vi "ConvertVariantToString.vi"(8 "error in":errorcluster, 10 "Variant":variant) -> (0 "error out":errorcluster, 1 "Array of VData":variant[](array[variant]), 2 "Variant dup":variant, 3 "String":string)   [LabVIEW 2012, in "Tree Tools.lvlib" / "Tree Tag Class.lvclass"]
uses:
  Tree Tag Class.lvclass
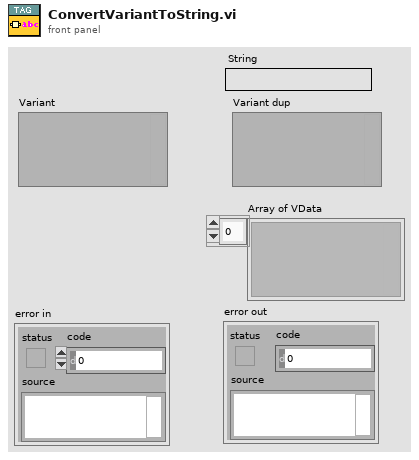
[diagram p1: front panel]
types:
  T1 = typedef "Type Descriptor Enumeration__ogtk.ctl" = enum8{"<Null>", "I8", "I16", "I32", "I64", "U8", "U16", "U32", "U64", "SGL", "DBL", "EXT", "CSG", "CDB", "CXT", "0x0F", "0x10", "0x11", "0x12", "0x13", "0x14", "Enum U8", "Enum U16", "Enum U32", "Enum U64", "SGL PQ", "DBL PQ", "EXT PQ", "CSG PQ", "CDB PQ", "CXT PQ", "0x1F", "0x20", "Boolean", "0x22", "0x23", "0x24", "0x25", "0x26", "0x27", "0x28", "0x29", "0x2A", "0x2B", "0x2C", "0x2D", "0x2E", "0x2F", "String", "0x31", "Path", "Pict", "0x34", "0x35", "0x36", "DAQ", "0x38", "0x39", "0x3A", "0x3B", "0x3C", "0x3D", "0x3E", "0x3F", "Array", "0x41", "0x42", "0x43", "0x44", "0x45", "0x46", "0x47", "0x48", "0x49", "0x4A", "0x4B", "0x4C", "0x4D", "0x4E", "0x4F", "Cluster", "0x51", "0x52", "Variant", "Waveform", "0x55", "0x56", "0x57", "0x58", "0x59", "0x5A", "0x5B", "0x5C", "0x5D", "0x5E", "0x5F", "0x60", "0x61", "0x62", "0x63", "0x64", "0x65", "0x66", "0x67", "0x68", "0x69", "0x6A", "0x6B", "0x6C", "0x6D", "0x6E", "0x6F", "Refnum"}
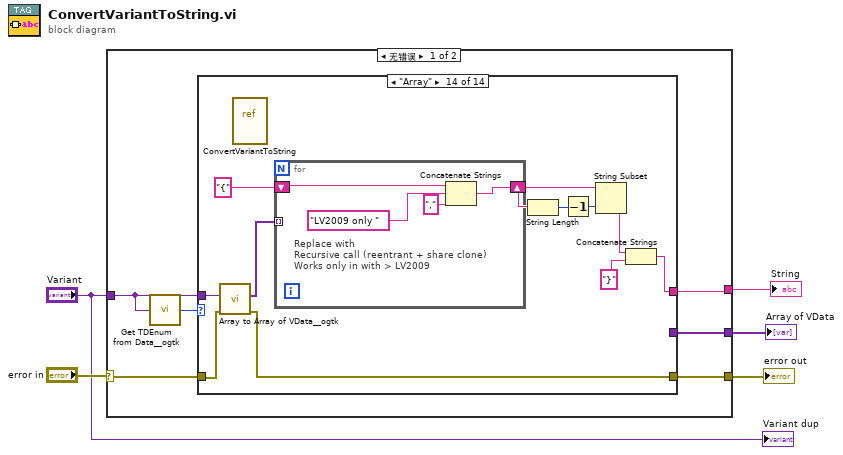
[diagram p0: block diagram]
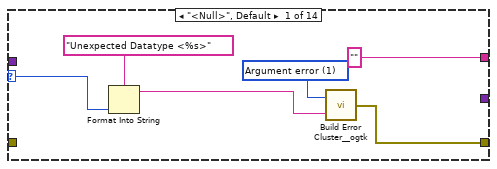
[diagram p2: hidden frame]
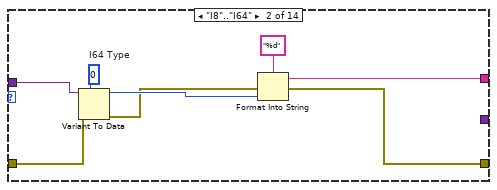
[diagram p3: hidden frame]
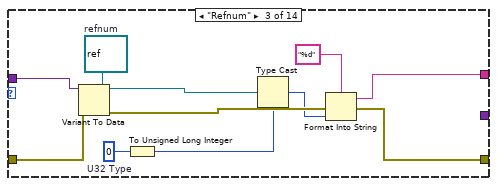
[diagram p4: hidden frame]
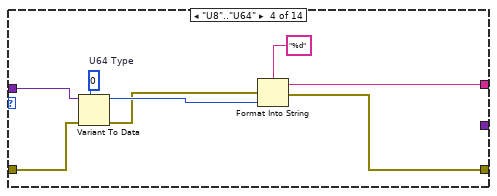
[diagram p5: hidden frame]
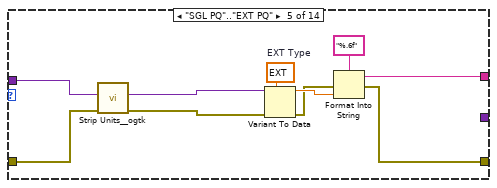
[diagram p6: hidden frame]
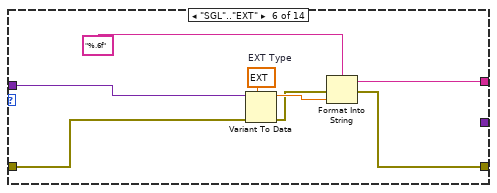
[diagram p7: hidden frame]
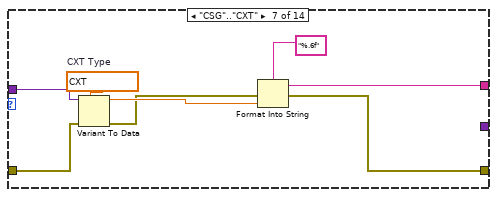
[diagram p8: hidden frame]
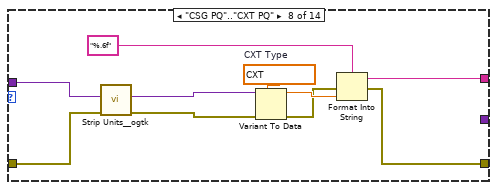
[diagram p9: hidden frame]
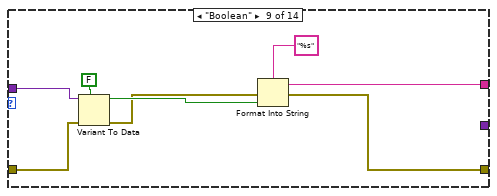
[diagram p10: hidden frame]
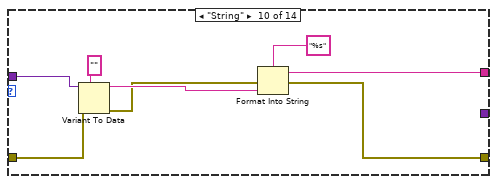
[diagram p11: hidden frame]
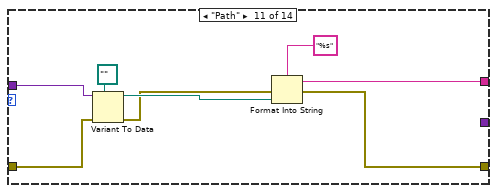
[diagram p12: hidden frame]
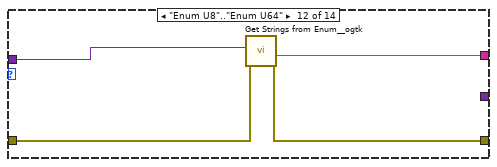
[diagram p13: hidden frame]
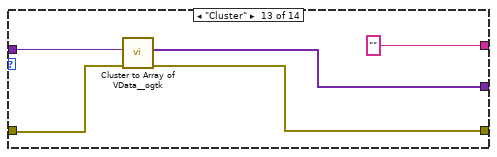
[diagram p14: hidden frame]
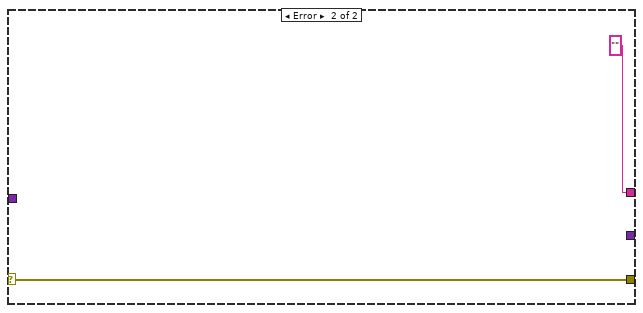
[diagram p15: hidden frame]
diagram:
  n1 = case shown="无错误" "error in" {
    selector: "error in" -> [w11 w130]
    tunnel: [w6 ""] -> w3
    tunnel: "Variant" -> [w9 _]
    tunnel: [w10 w130] -> w5
    tunnel: [w7 _] -> w1
    frame No Error {
      n2 = call <userlib>:"Get TDEnum from Data__ogtk.vi"("Data"=w9) -> ("Type Descriptor Enumeration"=w8:T1)  [unwired: 4 in]
      n3 = case shown="\"Array\"" w8 {
        selector: w8 -> [w13 _ _ _ _ _ _ _ _ _ _ _ _ _]
        tunnel: w9 -> [_ w24 w35 w43 w48 w57 w69 w74 w88 w96 w104 w108 w112 w124]
        tunnel: ["" w22 w33 w41 w52 w60 w67 w78 w86 w94 w102 w106 "" ("String Value") w114] -> w6
        tunnel: [w12 w19 w30 w38 w50 w58 w64 w76 w82 w91 w98 w105 w109 w122] -> w10
        tunnel: w11 -> [_ w21 w32 w40 w47 w56 w66 w73 w84 w90 w100 w107 w110 w123]
        tunnel: [_ _ _ _ _ _ _ _ _ _ _ _ w111 _] -> w7
        frame "<Null>", Default {
          w16 = 1 items=["No error", "Argument error", "Memory is full", "Out of zone", "End of file", "File already open", "Generic file I/O error", "File not found", "File permission error", "Disk is full", "Duplicate path", "Too many files open", "System feature not enabled", "Resource file not found", "Cannot add resource", "Resource not found", "Image not found", "Image memory error", "Pen does not exist", "Config type invalid", "Config token not found", "Config parse error", "Config memory error", "Bad external code format", "Bad external code offset", "External code not present", "Null window", "Destroy window error", "Null menu", "Print aborted", "Bad print record", "Print driver error", "Windows error during printing", "Memory error during printing", "Print dialog error", "Generic print error", "Invalid device refnum", "Device not found", "Device parameter error", "Device unit error", "Cannot open device", "Device call aborted", "Generic error", "Cancelled by user", "Object ID too low", "Object ID too high", "Object not in heap", "Unknown heap", "Unknown object (invalid DefProc)", "Unknown object (DefProc not in table)", "Message out of range", "Invalid (null) method", "Unknown message", "Manager call not supported", "Bad address", "Network operation in progress", "Network operation timed out", "Connection is busy", "Network attribute not supported", "Network error", "Address in use", "System out of memory", "Connection aborted", "Connection refused", "Not connected", "Already connected", "Connection closed", "Initialization error (interapplication manager)", "Bad occurrence", "Wait on unbound occurrence handler", "Occurrence queue overflow", "Datalog type conflict", "Unused", "Unrecognized type (interapplication manager)", "Memory corrupt", "Failed to make temporary DLL", "Old CIN version", "Drag socket not found", "Failed to load drop-object", "Failed to register OLE object", "Failed to release OLE object", "Format specifier type mismatch", "Unknown format specifier", "Too few format specifiers", "Too many format specifiers", "Scan failed", "Newer CIN version", "Error converting to variant", "Runtime menu error", "Password tampered", "Variant attribute not found", "Incompatible variant data type", "Event data is not available", "Event Store is not present", "Occurrence is not found", "Event Queue is not created", "Event info is not available", "Refnum passed is NULL", "Error retrieving Class GUID", "Error retrieving CoClass GUID", "Error retrieving TypeLib GUID.", "Bad built application magic bytes.", "Specific driver is different from the specific driver associated with the Logical Name.", "There is no session opened to the class driver.", "Max Error", "MAX - Error with config objects", "MAX - Error loading configuration", "MAX - Group not supported"]
          n4 = Format Into String(format string="Unexpected Datatype <%s>" ("Format String"), w13) -> (resulting string=w14:string)  [unwired: 2 in, 1 out]
          n5 = call <userlib>:"Build Error Cluster__ogtk.vi"("String to Prepend to source (\"\")"=w14, "code"=w16) -> ("error out"=w12:errorcluster)
        }
        frame "I8".."I64" {
          w25 = i64 0  # I64 Type
          n6 = Variant To Data(error in=w21, type=w25, Variant=w24) -> (data=w23:i64, error out=w20:errorcluster)
          n7 = Format Into String(format string="%d" ("name"), error in=w20, w23) -> (resulting string=w22:string, error out=w19:errorcluster)  [unwired: 1 in]
        }
        frame "Refnum" {
          w28 = u32 0  # U32 Type
          w36 = refnum<k0> refnum  # refnum
          n8 = Variant To Data(error in=w32, type=w36, Variant=w35) -> (data=w34:refnum<k0>, error out=w31:errorcluster)
          n9 = To Unsigned Long Integer(number=w28) -> (unsigned 32bit integer=w27:u32)
          n10 = Type Cast(type=w27, x=w34) -> (*(type *) &x=w29:u32)
          n11 = Format Into String(format string="%d" ("name"), error in=w31, w29) -> (resulting string=w33:string, error out=w30:errorcluster)  [unwired: 1 in]
        }
        frame "U8".."U64" {
          w44 = u64 0  # U64 Type
          n12 = Variant To Data(error in=w40, type=w44, Variant=w43) -> (data=w42:u64, error out=w39:errorcluster)
          n13 = Format Into String(format string="%d" ("name"), error in=w39, w42) -> (resulting string=w41:string, error out=w38:errorcluster)  [unwired: 1 in]
        }
        frame "SGL PQ".."EXT PQ" {
          w54 = ext 0.0  # EXT Type
          n14 = call <userlib>:"Strip Units__ogtk.vi"("error in (no error)"=w47, "Number or 1D array with units"=w48) -> ("error out"=w46:errorcluster, "Pure Number(s) (base units)"=w49:variant)  [unwired: 8 out]
          n15 = Variant To Data(error in=w46, type=w54, Variant=w49) -> (data=w53:ext, error out=w51:errorcluster)
          n16 = Format Into String(format string="%.6f" ("name"), error in=w51, w53) -> (resulting string=w52:string, error out=w50:errorcluster)  [unwired: 1 in]
        }
        frame "SGL".."EXT" {
          w62 = ext 0.0  # EXT Type
          n17 = Variant To Data(error in=w56, type=w62, Variant=w57) -> (data=w61:ext, error out=w59:errorcluster)
          n18 = Format Into String(format string="%.6f" ("name"), error in=w59, w61) -> (resulting string=w60:string, error out=w58:errorcluster)  [unwired: 1 in]
        }
        frame "CSG".."CXT" {
          w70 = cxt 0.0+0.0i  # CXT Type
          n19 = Variant To Data(error in=w66, type=w70, Variant=w69) -> (data=w68:cxt, error out=w65:errorcluster)
          n20 = Format Into String(format string="%.6f" ("name"), error in=w65, w68) -> (resulting string=w67:string, error out=w64:errorcluster)  [unwired: 1 in]
        }
        frame "CSG PQ".."CXT PQ" {
          w80 = cxt 0.0+0.0i  # CXT Type
          n21 = call <userlib>:"Strip Units__ogtk.vi"("error in (no error)"=w73, "Number or 1D array with units"=w74) -> ("error out"=w72:errorcluster, "Pure Number(s) (base units)"=w75:variant)  [unwired: 8 out]
          n22 = Variant To Data(error in=w72, type=w80, Variant=w75) -> (data=w79:cxt, error out=w77:errorcluster)
          n23 = Format Into String(format string="%.6f" ("name"), error in=w77, w79) -> (resulting string=w78:string, error out=w76:errorcluster)  [unwired: 1 in]
        }
        frame "Boolean" {
          n24 = Variant To Data(error in=w84, type=FALSE, Variant=w88) -> (data=w87:bool, error out=w83:errorcluster)
          n25 = Format Into String(format string="%s" ("name"), error in=w83, w87) -> (resulting string=w86:string, error out=w82:errorcluster)  [unwired: 1 in]
        }
        frame "String" {
          n26 = Variant To Data(error in=w90, type="", Variant=w96) -> (data=w95:string, error out=w92:errorcluster)
          n27 = Format Into String(format string="%s" ("name"), error in=w92, w95) -> (resulting string=w94:string, error out=w91:errorcluster)  [unwired: 1 in]
        }
        frame "Path" {
          n28 = Variant To Data(error in=w100, type=path "", Variant=w104) -> (data=w103:path, error out=w99:errorcluster)
          n29 = Format Into String(format string="%s" ("name"), error in=w99, w103) -> (resulting string=w102:string, error out=w98:errorcluster)  [unwired: 1 in]
        }
        frame "Enum U8".."Enum U64" {
          n30 = call <userlib>:"Get Strings from Enum__ogtk.vi"("error in (no error)"=w107, "Enum"=w108) -> ("error out"=w105:errorcluster, "String Value"=w106:string)  [unwired: 8 out]
        }
        frame "Cluster" {
          n31 = call <userlib>:"Cluster to Array of VData__ogtk.vi"("error in (no error)"=w110, "Cluster"=w112) -> ("error out"=w109:errorcluster, "Array of VData"=w111:variant[])  [unwired: 8 out]
        }
        frame "Array" {
          n32 = call <userlib>:"Array to Array of VData__ogtk.vi"("error in (no error)"=w123, "MultiD Array"=w124) -> ("error out"=w122:errorcluster, "1D Array of Variants"=w121:variant[])  [unwired: 8 out]
          n33 = vi-ref "ConvertVariantToString.vi"() -> ()  [unwired: 1 out]
          n34 = for {
            tunnel: w121 -> [_] mode=indexing
            shift-right: [w126] -> w119
            shift-left: "{" ("String Value") -> [w128]
            # "Replace with \nRecursive call (reentrant + share clone)\nWorks only in with > LV2009"
            n35 = Concatenate Strings(w128, "LV2009 only " ("string"), "," ("string")) -> (w126:string)
          }
          n36 = String Length(string=w119) -> (length=w118:i32)
          n37 = Decrement(x=w118) -> (x-1=w117:i32)
          n38 = String Subset(string=w119, length (rest)=w117) -> (substring=w116:string)  [unwired: 1 out]
          n39 = Concatenate Strings(w116, "}" ("String Value")) -> (w114:string)
        }
      }
    }
    frame Error {
    }
  }
  "error out" <- w5
  "String" <- w3
  "Array of VData" <- w1
  "Variant dup" <- "Variant"
